vi "server health check.vi"(8 "error in":errorcluster) -> (0 "error out":errorcluster, 3 "healthy":bool)   [LabVIEW 2024]
uses:
  <vilib>/httpClient/LabVIEWHTTPClient.lvlib
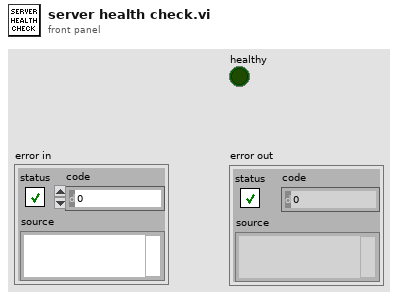
[diagram p1: front panel]
types:
  T1 = typedef "LabVIEWHTTPClient.lvlib/ClientHandle.ctl" = refnum<k1>
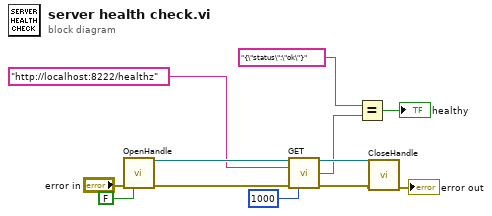
[diagram p0: block diagram]
diagram:
  n1 = call <vilib>:"OpenHandle.vi"("error in (no error)"="error in", "verify server(true)"=FALSE) -> ("client handle out"=w12:T1, "error out"=w11:errorcluster)  [unwired: 12 in]
  n2 = call <vilib>:"GET.vi"("client handle"=w12, "url"="http://localhost:8222/healthz", "error in (no error)"=w11, "timeout (10000)"=1000) -> ("client handle out"=w8:T1, "body"=w4:string, "error out"=w7:errorcluster)  [unwired: 8 in, 1 out]
  n3 = Equal?(x="{\"status\":\"ok\"}", y=w4) -> (x = y?=→"healthy":bool)
  n4 = call <vilib>:"CloseHandle.vi"("client handle"=w8, "error in (no error)"=w7) -> ("error out"=→"error out":errorcluster)  [unwired: 13 in]
